vi "Write name.vi"(8 "error in (no error)":errorcluster, 10 "name":string, 11 "DAQmxTask in":refnum<class "DAQmxTask.lvclass">) -> (0 "error out":errorcluster, 3 "DAQmxTask out":refnum<class "DAQmxTask.lvclass">)   [LabVIEW 2019, in "DAQmxTask.lvclass"]
uses:
  DAQmxTask.lvclass
  DAQmxTask.lvclass/DAQmxTask.ctl
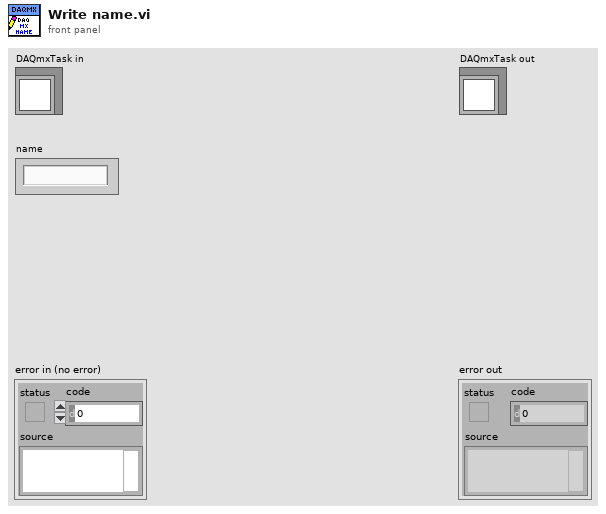
[diagram p1: front panel]
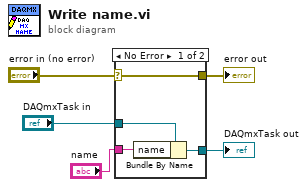
[diagram p0: block diagram]
diagram:
  n1 = case shown="No Error" "error in (no error)" {
    selector: "error in (no error)" -> [w9 w10]
    tunnel: [w9 w10] -> w4
    tunnel: [w7 w11] -> w2
    tunnel: "DAQmxTask in" -> [w8 w11]
    tunnel: "name" -> [w6 _]
    frame No Error {
      n2 = Bundle By Name(cluster=w8, "name"=w6) -> (w7:refnum<class "DAQmxTask.lvclass">)
    }
    frame Error {
    }
  }
  "error out" <- w4
  "DAQmxTask out" <- w2
